vi "Time64 to Timestamp.vi"(1 "Time64 In":u64) -> (0 "Time Stamp":timestamp)   [LabVIEW 2009, in "Time.lvlib"]
uses:
  Time.lvlib
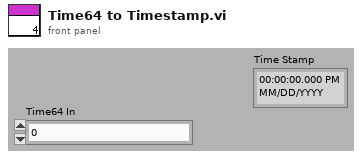
[diagram p1: front panel]
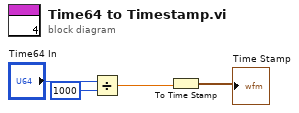
[diagram p0: block diagram]
diagram:
  n1 = Divide(x="Time64 In", y=u64 1000) -> (x/y=w2:dbl)
  n2 = To Time Stamp(1:w2) -> (0:→"Time Stamp":timestamp)
